vi "Close Serial.vi"() -> ()   [LabVIEW 2019]
panel:
  out "error out":errorcluster
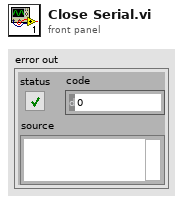
[diagram p1: front panel]
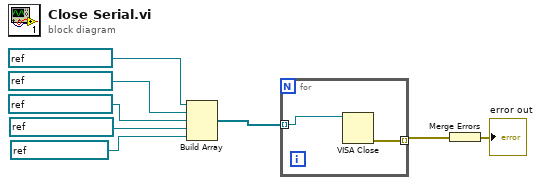
[diagram p0: block diagram]
diagram:
  n1 = Build Array(refnum<visa-resource-name> "ASRL10::INSTR" ("VISA resource name"), refnum<visa-resource-name> "ASRL11::INSTR" ("VISA resource name"), refnum<visa-resource-name> "ASRL12::INSTR" ("VISA resource name"), refnum<visa-resource-name> "ASRL13::INSTR" ("VISA resource name"), refnum<visa-resource-name> "ASRL1::INSTR" ("VISA resource name")) -> (w3:refnum<visa-resource-name>[])
  n2 = for {
    tunnel: w3 -> [w10] mode=indexing
    tunnel: [w9] -> w2 mode=indexing
    n3 = VISA Close(VISA resource name=w10) -> (error out=w9:errorcluster)  [unwired: 1 in]
  }
  n4 = Merge Errors(w2) -> (→"error out":errorcluster)
